vi "dataProcess_peaks_extended.vi"(0 "reference":refnum<class "OSA.lvclass">, 1 "X search full range":bool=TRUE, 7 "error in (no error)":errorcluster, 8 "X search min (/cm)":sgl format="%.2f", 9 "minPeakHeight (dB)":sgl format="%.2f", 12 "X search max (/cm)":sgl format="%.2f", 13 "thld (mW)":sgl format="%.2f", 15 "sorting (none)":enum16{"none", "position", "height", "width"}(ring)) -> (16 "peaks thld left":sgl[](array[numeric]), 17 "peakCenter centroid, (wavenr/cm)":sgl[](array[numeric]) format="%.2f", 18 "peaks thld right":sgl[](array[numeric]), 19 "peakHeight centroid, (mW power absolute)":sgl[](array[numeric]) format="%.2f", 20 "duplicate reference":refnum<class "OSA.lvclass">, 21 "nr peaksFound":i32, 23 "peak position, (wavenr/cm)":sgl[](array[numeric]) format="%.2f", 24 "peakWidth, (wavenr/cm)":sgl[](array[numeric]) format="%.2f", 25 "peakHeight, (mW power absolute)":sgl[](array[numeric]) format="%.2f", 27 "error out":errorcluster)   [LabVIEW 2010, in "OSA.lvclass"]
doc: "Make use of FTSLib FTS_FindPeaks_ext which enable a more detailed peaks characterisation, (centroid algorithm)."
uses:
  OSA.lvclass
  typeDef/spectrum_y_unit.ctl
  FTSLib.dll
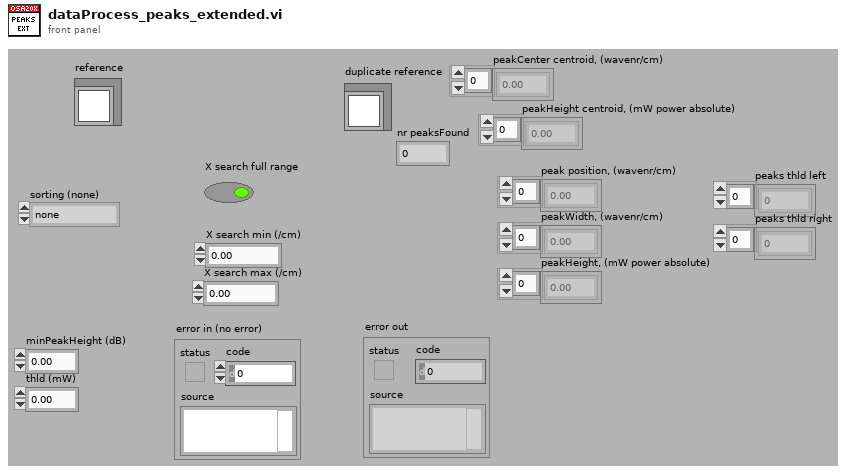
[diagram p1: front panel]
types:
  T1 = typedef "OSA.lvclass/spectrum_y_unit.ctl" = enum16{"dBm pwr absolute", "dBm pwr density", "mW pwr absolute", "mW pwr density"}
  T2 = enum16{"get", "init", "set interferogram", "set spectrum", "cleanUp"}
  T3 = typedef "OSA.lvclass/ObjectAttributes.ctl" = cluster{"Stop":bool, "dataType":T4, "spectrometerIdx":u16, "buffer size interferogram":i32, "interferogram":cluster{"new":bool, "plot_x_ min":sgl, "plot_x_max":sgl, "plot_y_min":sgl, "plot_y_max":sgl, "Graph Intrfrgrm":T5, "timeStamp":u32, "signal (%)":dbl, "traces":cluster{"idx":u32, "broadBand":bool, "monoChromatic":bool, "peakToPeakSignal":dbl, "peakToPeakPos":dbl}[], "traces idx last":i32}, "spectrum":cluster{"new":bool, "plot_x_min":sgl, "plot_x_max":sgl, "plot_unit_x":T6, "plot_unit_y":T7, "plot_y_min":sgl, "plot_y_max":sgl, "Graph Spectrum":T5, "timeStamp":u32, "X_VAL_OPTIONS":enum16{"MIN_MAX", "ARRAY"}, "traces":cluster{"idx":u32}[], "traces idx last":i32}, "Thorlabs_OSA_64.lvclass:queue_action.ctlqueue ref":refnum<queue>, "action":T8, "plot zoom step":dbl, "buffer semaphore":T9, "acq stopped":bool, "dataType active":T4, "temperature (degr C)":sgl, "pressure (hPa)":sgl, "rel humidity (%)":sgl, "settings":cluster{"resolution":T10, "sensitivity":T11, "Average":bool, "average nr":u32, "apodisation":T12, "acq delay (ms)":u32, "airMesure":T13, "wmtr on":bool, "intfgrm_smooth_width":u16, "intfgrm_smooth_nrOfPasses":u16, "intfgrm_smooth":T14, "phaseCorrection":T15, "zeroFill":u8, "spectr_smooth":T14, "spectr_smooth_width":u16, "spectr_smooth_nrOfPasses":u16, "resolution (/cm)":sgl, "REF wavelength, (nm)":dbl, "gain_idx":u16, "gainAuto":bool, "gain_relative":dbl, "PD sensitivity mode":T16, "PD senseMode implemented":bool, "SensorTemperature implemented":bool, "SensorPressure implemented":bool, "SensorHumidity implemented":bool}, "peaks position":sgl[], "peaks width":sgl[], "peaks height":sgl[], "peaks max nr":u32, "peaks latest nr":i32, "peaks new":bool, "power":dbl, "power new":bool, "path":string, "wavelength (WNr)":dbl, "wavelength new":bool, "buffer size spectrum":i32, "status":string, "VI reference":refnum<vi>, "funcPointer":u64, "libraryPointer":u64, "singleAcquisition":bool, "coherenceLength (cm)":dbl, "coherenceLength new":bool, "spectrometer model":string, "spectrometer serial nr":string, "peaks thld left":sgl[], "peaks thld right":sgl[], "coherenceLength error (cm)":dbl, "ADC bits":u16, "peaks position centroid":sgl[], "peaks height centroid":sgl[], "OSA series":T17, "channel index spectrum":u16, "spectrometer rangeLow, (/cm)":dbl, "spectrometer rangeHigh, (/cm)":dbl, "channel index interferogram":u16}
  T4 = typedef "OSA.lvclass/acq_dataType.ctl" = enum16{"none", "interferogram", "spectrum"}
  T5 = typedef "OSA.lvclass/graph_intensity.ctl" = refnum<vi>
  T6 = typedef "OSA.lvclass/spectrum_x_unit.ctl" = enum16{"wavenr/cm", "THz", "eV", "nm_air", "nm_vac"}
  T7 = typedef "OSA.lvclass/y_unit.ctl" = enum16{"ADC counts", "dBm pwr absolute", "dBm pwr density", "mW pwr absolute", "mW pwr density"}
  T8 = typedef "OSA.lvclass/queue_action.ctl" = enum16{"none", "stop", "GUI_plotInterferogram", "GUI_plotSpectrum", "GUI_plotInterferogramRescale", "GUI_plotSpectrumRescale", "GUI_plotInterferogramReset", "GUI_plotSpectrumReset", "GUI_plotInterferogramAutoScaleY", "GUI_plotSpectrumAutoScaleY", "GUI_plotInterferogramZoomOut", "GUI_plotSpectrumZoomOut", "GUI_plotInterferogramPane", "GUI_plotSpectrumPane", "GUI_plotInterferogramZoomMouse", "GUI_plotSpectrumZoomMouse", "ENVIRONMENT temperature", "ENVIRONMENT pressure", "MODE_resolution set", "MODE_resolution get", "MODE_sensitivity set", "MODE_sensitivity get", "MODE_PDTemperature set", "MODE_PDTemperature get", "REBOOT/RESET firmware", "ACQASYNC_acquireSingleSpectrum", "ACQASYNC_continuous start", "ACQASYNC_continuous stop\n", "ACQASYNC_get last interferogram", "ACQASYNC_get last spectrum", "ACQASYNC_get last waveNr", "ACQOPT_interferogram smoothing set", "ACQOPT_interferogram smoothing get", "ACQOPT_spectrum smoothing set", "ACQOPT_spectrum smoothing get", "ACQOPT_apodisation type set", "ACQOPT_apodisation type get", "ACQOPT_phase correction type set", "ACQOPT_phase correction type get", "ACQOPT_acqIntervall_set", "ACQOPT_acqIntervall_get", "ACQOPT_average spectrum set", "ACQOPT_average spectrum get", "ACQOPT_rolling average set", "ACQOPT_rolling average get", "ACQOPT_zero fill factor set", "ACQOPT_zero fill factor get", "ACQOPT_cycle counting set", "ACQOPT_cycle counting get", "ACQOPT_air measure option set", "ACQOPT_air measure option get", "ACQOPT_gainLevel auto get", "ACQOPT_gainLevel auto set", "ACQOPT_gainLevel get", "ACQOPT_gainLevel set", "ACQOPT_getAll", "INSTRUMENT_PROPERTY_range_WaveNr_min", "INSTRUMENT_PROPERTY_range_WaveNr_max", "INSTRUMENT_PROPERTY_reference_wavelength_cm^-1", "INSTRUMENT_PROPERTY_samplesPerRefPeriod", "INSTRUMENT_PROPERTY_resolution_waveNrPercm", "INSTRUMENT_PROPERTY_availableGainLevels", "INSTRUMENT_PROPERTY_status", "CONVERT", "ANALYSE_POWER", "ANALYSE_PEAKS", "ANALYSE_WAVELENGTH", "ANALYSE_SPECTRUM", "ANALYSE_INTERFEROGRAM", "ANALYSE_COHERENCE_LENGTH", "MATH", "MATH_power", "MATH_peaks", "FILE", "miscellaneous"}
  T9 = typedef "Semaphore RefNum" = refnum<k1>
  T10 = typedef "OSA.lvclass/resolution.ctl" = enum16{"low", "high"}
  T11 = typedef "OSA.lvclass/sensitivityMode.ctl" = enum16{"low", "low medium", "high medium", "high"}
  T12 = typedef "OSA.lvclass/apodisation.ctl" = enum16{"NONE", "NORTON_BEER_WEAK", "NORTON_BEER_MEDIUM", "NORTON_BEER_STRONG", "TRIANGULAR", "COSINE", "HANN", "HAMMING", "BLACKMANHARRIS3", "BLACKMANHARRIS4", "GAUSSIAN"}
  T13 = typedef "OSA.lvclass/airMeasure.ctl" = enum16{"TEMPERATURE", "PRESSURE"}
  T14 = typedef "OSA.lvclass/interferogram_smoothing.ctl" = enum16{"NONE", "BINOMIAL", "SAVITSKY_GOLAY", "FOURIER", "MOVING_AVERAGE", "GAUSSIAN"}
  T15 = typedef "OSA.lvclass/phaseCorrection.ctl" = enum16{"NONE", "MERTZ", "FORMAN", "MERTZ_FILE", "FORMAN_FILE", "FUTURE COMP."}
  T16 = typedef "OSA.lvclass/PDTemperatureMode.ctl" = enum16{"cool: better sensitivity/noise floor", "warm: extended wl range"}
  T17 = typedef "OSA.lvclass/OSA_series.ctl" = enum16{"OSA200", "OSA300", "UNKNOWN"}
  T18 = typedef "OSA20X.lvclass/xVal_option.ctl" = enum16{"MIN_MAX", "ARRAY"}
  T19 = cluster{"length":u32, "X min":sgl, "X max":sgl, "X_VAL_OPTIONS":T18}
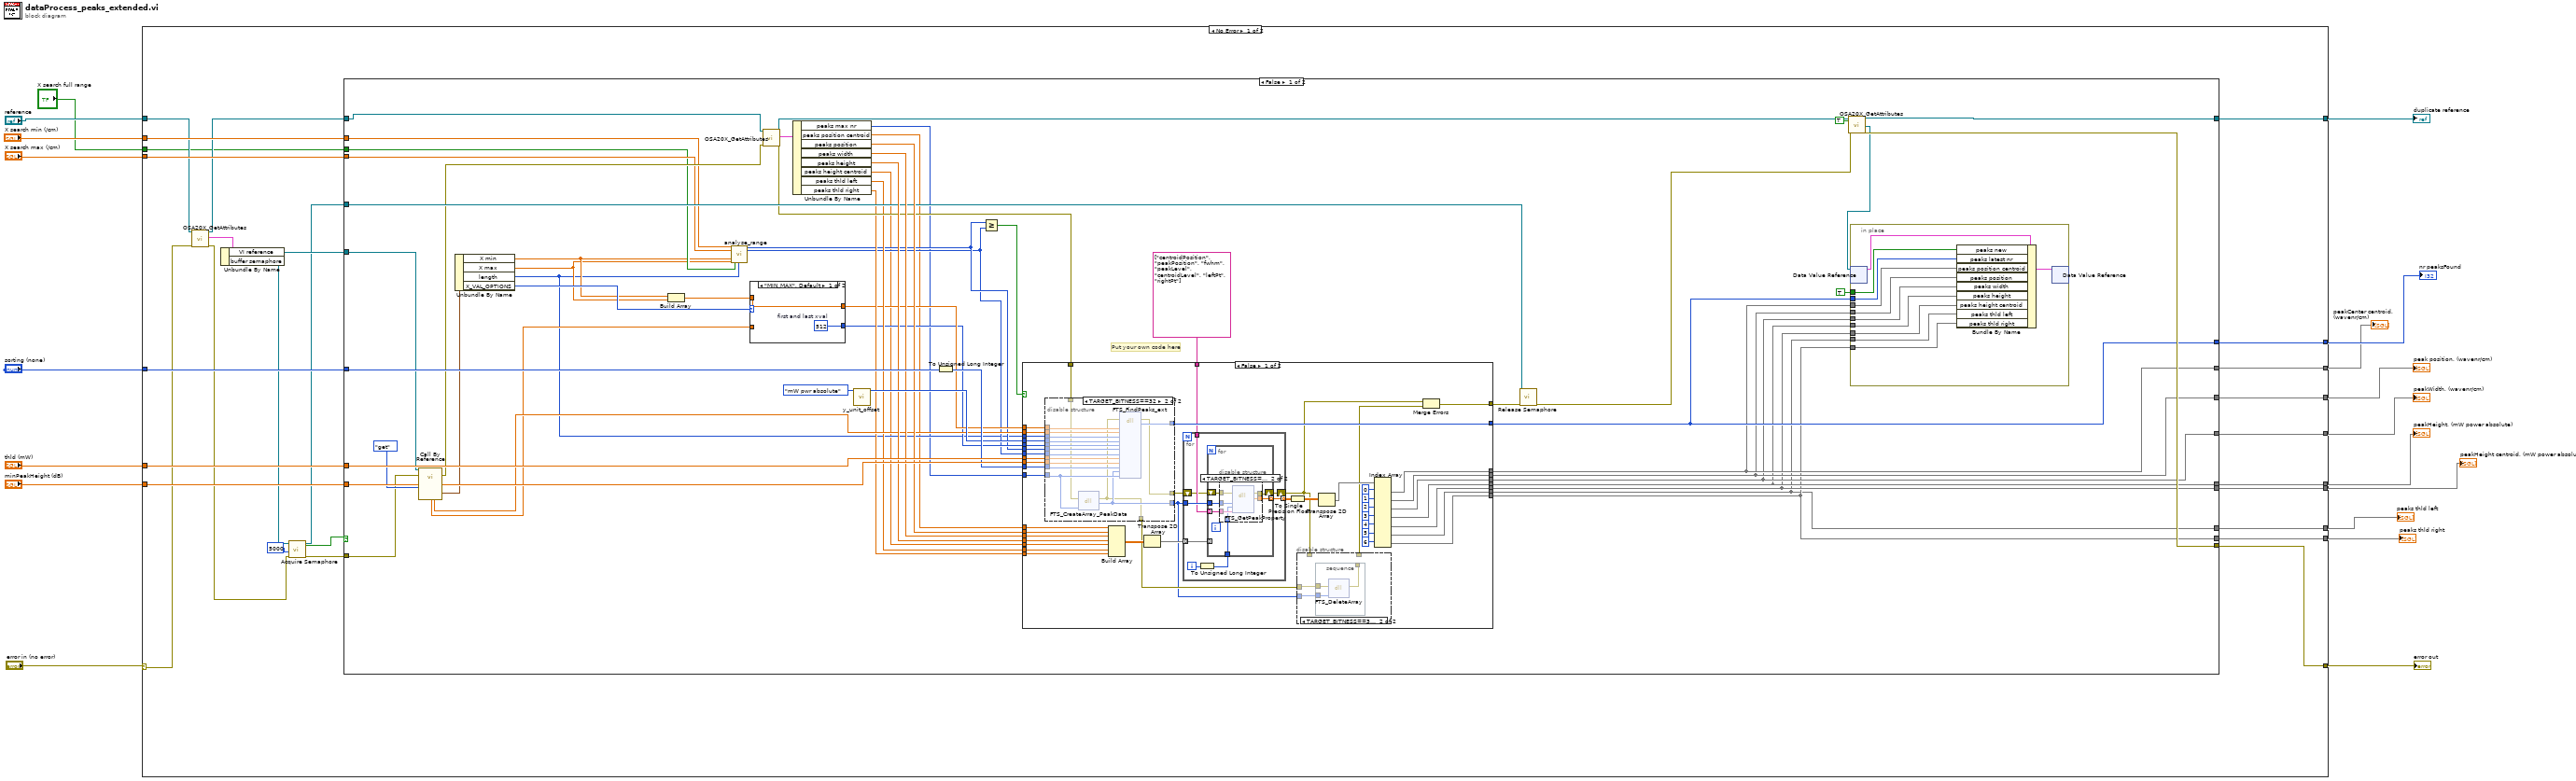
[diagram p0: block diagram]
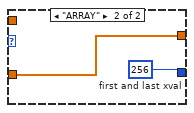
[diagram p2: hidden frame]
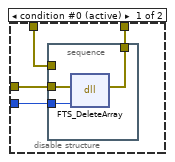
[diagram p3: hidden frame]
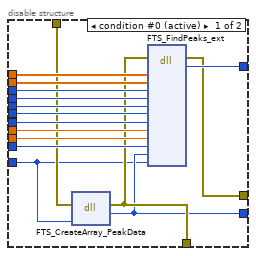
[diagram p4: hidden frame]
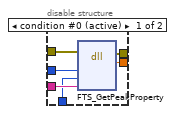
[diagram p5: hidden frame]
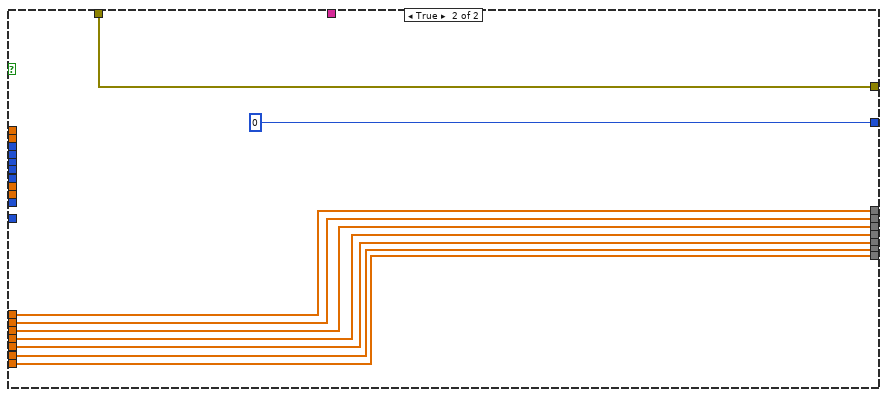
[diagram p6: hidden frame]
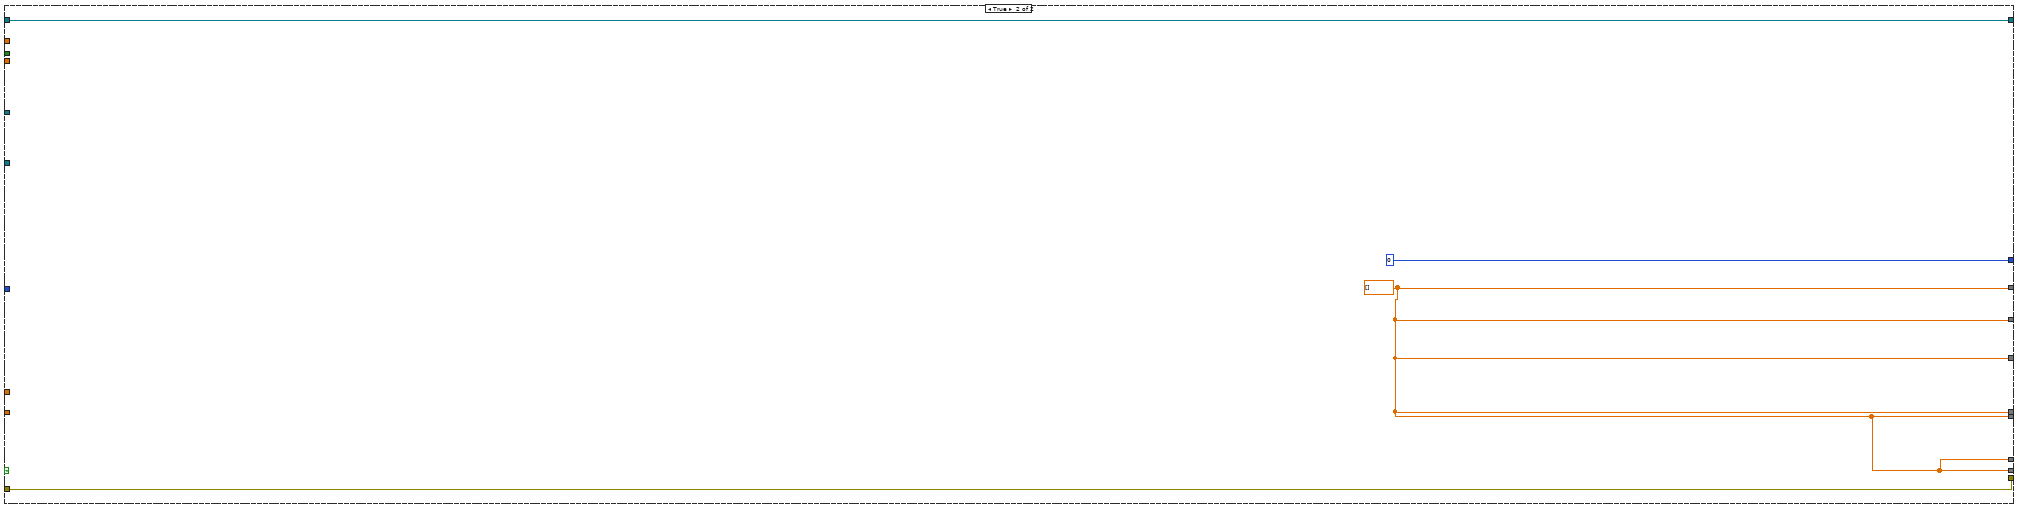
[diagram p7: hidden frame]
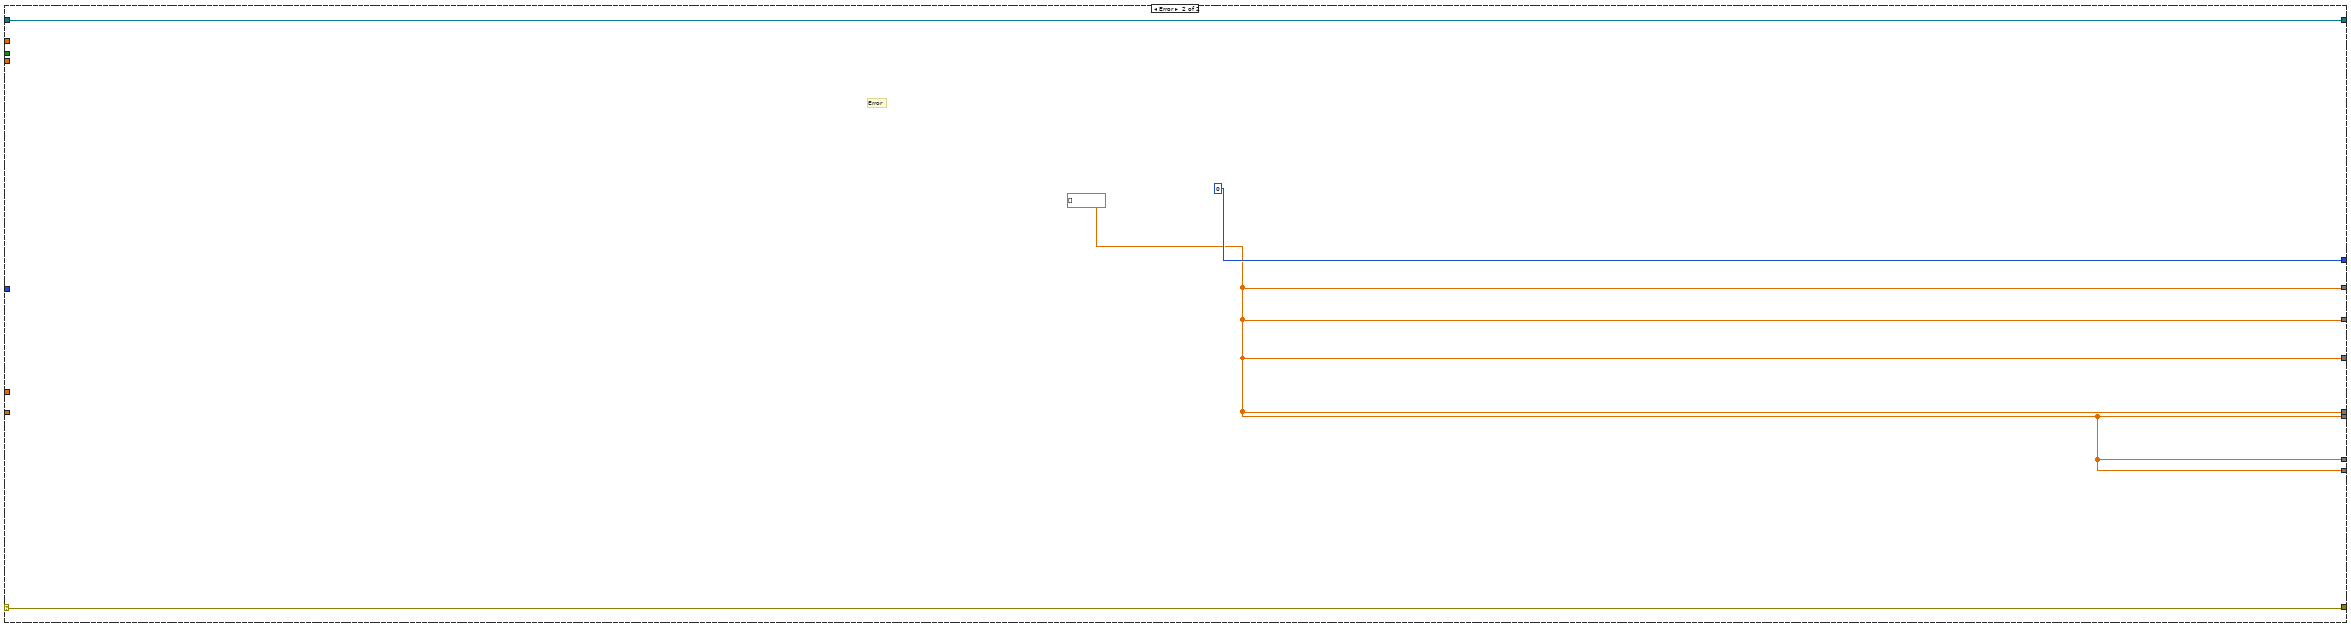
[diagram p8: hidden frame]
diagram:
  n1 = case shown="No Error" "error in (no error)" {
    selector: "error in (no error)" -> [w33 w247]
    tunnel: [w41 w247] -> w18
    tunnel: "reference" -> [w27 w248]
    tunnel: [w42 w248] -> w15
    tunnel: "minPeakHeight (dB)" -> [w45 _]
    tunnel: "thld (mW)" -> [w44 _]
    tunnel: "sorting (none)" -> [w43 _]
    tunnel: [w38 w245] -> w5
    tunnel: [w37 w245] -> w4
    tunnel: [w39 w245] -> w3
    tunnel: [w40 0] -> w11
    tunnel: "X search min (/cm)" -> [w36 _]
    tunnel: "X search max (/cm)" -> [w35 _]
    tunnel: [w23 w245] -> w2
    tunnel: [w22 w245] -> w1
    tunnel: "X search full range" -> [w21 _]
    tunnel: [w20 w245] -> w7
    tunnel: [w19 w245] -> w6
    frame No Error {
      n2 = call "OSA20X_GetAttributes.vi"("reference in"=w27, "error in (no error)"=w33) -> ("reference out"=w26:refnum<class "OSA.lvclass">, "Data"=w24:T3, "error out"=w32:errorcluster)  [unwired: 14 in, 1 out]
      n3 = Unbundle By Name(w24) -> ("VI reference"=w28:refnum<vi>, "buffer semaphore"=w30:T9)
      n4 = call <vilib>:"Acquire Semaphore.vi"("error in (no error)"=w32, "ms timeout (-1)"=5000, "semaphore"=w30) -> ("error out"=w31:errorcluster, "timed out"=w29:bool, "semaphore out"=w25:T9)  [unwired: 2 in]
      n5 = case shown="False" w29 {
        tunnel: w45 -> [w100 _]
        tunnel: w44 -> [w99 _]
        tunnel: w43 -> [w98 _]
        tunnel: w26 -> [w97 w243]
        tunnel: [w94 w243] -> w42
        tunnel: [w93 w242] -> w41
        tunnel: [w74 0 ("return type")] -> w40
        tunnel: [w71 w241] -> w39
        tunnel: [w73 w241] -> w38
        tunnel: [w72 w241] -> w37
        tunnel: w36 -> [w58 _]
        tunnel: w35 -> [w57 _]
        tunnel: w31 -> [w86 w242]
        tunnel: w28 -> [w85 _]
        tunnel: w25 -> [w80 _]
        tunnel: [w67 w241] -> w23
        tunnel: [w66 w241] -> w22
        tunnel: w21 -> [w56 _]
        tunnel: [w47 w241] -> w20
        tunnel: [w46 w241] -> w19
        frame False {
          # "Put your own code here"
          n6 = call-by-ref "?"(reference=w85, error in=w86, "action"=T2."get") -> (error out=w79:errorcluster, "spectrum X"=w64:sgl[], "spectrum Y"=w84:sgl[], "spectrum property"=w83:T19)  [unwired: 14 in, 3 out]
          n7 = Unbundle By Name(w83) -> ("X min"=w54:sgl, "X max"=w53:sgl, "length"=w52:u32, "X_VAL_OPTIONS"=w61:T18)
          n8 = Build Array(w54, w53) -> (w55:sgl[])
          n9 = call "analyse_range.vi"("X search min (/cm)"=w58, "X search max (/cm)"=w57, "X min"=w54, "X max"=w53, "full range"=w56, "length"=w52) -> ("index start"=w60:u32, "index stop"=w59:u32)  [unwired: 12 in]
          n10 = case shown="\"MIN_MAX\", Default" w61 {
            tunnel: w64 -> [_ w104]
            tunnel: [w102 w104] -> w63
            tunnel: w55 -> [w102 _]
            tunnel: [w101 w103] -> w62
            frame "MIN_MAX", Default {
              w101 = u32 512  # first and last xval
            }
            frame "ARRAY" {
              w103 = u32 256  # first and last xval
            }
          }
          n11 = call "OSA20X_GetAttributes.vi"("reference in"=w97, "error in (no error)"=w79) -> ("reference out"=w95:refnum<class "OSA.lvclass">, "Data"=w77:T3, "error out"=w70:errorcluster)  [unwired: 14 in, 1 out]
          n12 = Unbundle By Name(w77) -> ("peaks max nr"=w51:u32, "peaks position centroid"=w50:sgl[], "peaks position"=w90:sgl[], "peaks width"=w89:sgl[], "peaks height"=w88:sgl[], "peaks height centroid"=w49:sgl[], "peaks thld left"=w69:sgl[], "peaks thld right"=w68:sgl[])
          n13 = call "y_unit_offset.vi"("spectrum y unit (mW pwr absolute)"=spectrum_y_unit."mW pwr absolute") -> ("yUnit val"=w92:i32)  [unwired: 18 in]
          n14 = To Unsigned Long Integer(number=w98) -> (unsigned 32bit integer=w96:u32)
          n15 = Greater Or Equal?(x=w60, y=w59) -> (x >= y?=w91:bool)
          n16 = case shown="False" w91 {
            tunnel: w100 -> [w161 _]
            tunnel: w99 -> [w160 _]
            tunnel: w96 -> [w159 _]
            tunnel: w90 -> [w147 w237]
            tunnel: w89 -> [w146 w236]
            tunnel: w88 -> [w145 w235]
            tunnel: w51 -> [w116 _]
            tunnel: [w158 0] -> w74
            tunnel: w84 -> [w157 _]
            tunnel: [w135 w236] -> w71
            tunnel: [w137 w238] -> w73
            tunnel: [w136 w237] -> w72
            tunnel: w92 -> [w156 _]
            tunnel: w62 -> [w155 _]
            tunnel: w63 -> [w154 _]
            tunnel: w52 -> [w153 _]
            tunnel: w60 -> [w152 _]
            tunnel: w59 -> [w151 _]
            tunnel: [w119 w239] -> w82
            tunnel: w70 -> [w150 w239]
            tunnel: w69 -> [w143 w233]
            tunnel: w68 -> [w142 w232]
            tunnel: [w134 w235] -> w67
            tunnel: [w133 w234] -> w66
            tunnel: w50 -> [w148 w238]
            tunnel: w49 -> [w144 w234]
            tunnel: string[] ["centroidPosition", "peakPosition", "fwhm", "peakLevel", "centroidLevel", "leftPt", "rightPt"] -> [w149 _]
            tunnel: [w125 w233] -> w46
            tunnel: [w124 w232] -> w47
            frame False {
              n17 = disable-structure shown="TARGET_BITNESS==32" {
                disable-tunnel: w161 -> [w189 w197]
                disable-tunnel: w160 -> [w188 w198]
                disable-tunnel: w159 -> [w187 w196]
                disable-tunnel: [w186 w193] -> w158
                disable-tunnel: w157 -> [w185 w204]
                disable-tunnel: w156 -> [w184 w202]
                disable-tunnel: w155 -> [w183 w201]
                disable-tunnel: w154 -> [w182 w205]
                disable-tunnel: w153 -> [w181 w203]
                disable-tunnel: w152 -> [w180 w200]
                disable-tunnel: w151 -> [w179 w199]
                disable-tunnel: w150 -> [w178 w194]
                disable-tunnel: [w177 w192] -> w122
                disable-tunnel: [w176 w190] -> w121
                disable-tunnel: [w175 w191] -> w117
                disable-tunnel: w116 -> [w174 w195]
                frame condition #0 (active) {
                  n18 = dll-call lib="FTSLib.dll" fn="FTS_CreateArray_PeakData"(error in=w178, "number"=w174) -> (error out=w176:errorcluster, "return type"=w175:u64)  [unwired: 3 in, 1 out]
                  n19 = dll-call lib="FTSLib.dll" fn="FTS_FindPeaks_ext"(error in=w176, "xData"=w182, "yData"=w185, "length"=w181, "yAxisUnit"=w184, "xValueOption"=w183, "idxStart"=w180, "idxStop"=w179, "thld"=w188, "minPeakHeight_dB"=w189, "option"=w187, "peakArray"=w175, "maxPeaks"=w174) -> (error out=w177:errorcluster, "return type"=w186:i32)  [unwired: 14 in, 1 out]
                }
                frame condition #1 {
                  n20 = dll-call lib="FTSLib.dll" fn="FTS_CreateArray_PeakData"(error in=w194, "number"=w195) -> (error out=w190:errorcluster, "return type"=w191:u32)  [unwired: 3 in, 1 out]
                  n21 = dll-call lib="FTSLib.dll" fn="FTS_FindPeaks_ext"(error in=w190, "xData"=w205, "yData"=w204, "length"=w203, "yAxisUnit"=w202, "xValueOption"=w201, "idxStart"=w200, "idxStop"=w199, "thld"=w198, "minPeakHeight_dB"=w197, "option"=w196, "peakArray"=w191, "maxPeaks"=w195) -> (error out=w192:errorcluster, "return type"=w193:i32)  [unwired: 14 in, 1 out]
                }
              }
              n22 = Build Array(w148, w147, w146, w145, w144, w143, w142) -> (w141:sgl[][])
              n23 = Transpose 2D Array(2D array=w141) -> (transposed array=w140:sgl[][])
              n24 = for {
                tunnel: w117 -> [w213]
                tunnel: w149 -> [w212]
                tunnel: w140 -> [w211] mode=indexing
                tunnel: [w208] -> w139 mode=indexing
                shift-right: [w206] -> w118
                shift-left: w122 -> [w207]
                i -> [w210]
                n25 = To Unsigned Long Integer(number=w210) -> (unsigned 32bit integer=w209:u32)
                n26 = for {
                  tunnel: w213 -> [w219]
                  tunnel: w212 -> [w218] mode=indexing
                  tunnel: w211 -> [_] mode=indexing
                  tunnel: [w217] -> w208 mode=indexing
                  tunnel: w209 -> [w216]
                  shift-right: [w214] -> w206
                  shift-left: w207 -> [w215]
                  n27 = disable-structure shown="TARGET_BITNESS==32" {
                    disable-tunnel: w219 -> [w225 w231]
                    disable-tunnel: w218 -> [w224 w228]
                    disable-tunnel: [w223 w226] -> w217
                    disable-tunnel: w216 -> [w222 w227]
                    disable-tunnel: w215 -> [w221 w230]
                    disable-tunnel: [w220 w229] -> w214
                    frame condition #0 (active) {
                      n28 = dll-call lib="FTSLib.dll" fn="FTS_GetPeakProperty"(error in=w221, "peakArray"=w225, "indexOfPeak"=w222, "parameterName"=w224) -> (error out=w220:errorcluster, "return type"=w223:dbl)  [unwired: 5 in, 1 out]
                    }
                    frame condition #1 {
                      n29 = dll-call lib="FTSLib.dll" fn="FTS_GetPeakProperty"(error in=w230, "peakArray"=w231, "indexOfPeak"=w227, "parameterName"=w228) -> (error out=w229:errorcluster, "return type"=w226:dbl)  [unwired: 5 in, 1 out]
                    }
                  }
                }
              }
              n30 = To Single Precision Float(number=w139) -> (single precision float=w123:sgl[][])
              n31 = disable-structure shown="TARGET_BITNESS==32" {
                disable-tunnel: w121 -> [w165 w169]
                disable-tunnel: [w164 _] -> w120
                disable-tunnel: w118 -> [w163 _]
                disable-tunnel: w117 -> [w162 w170]
                frame condition #0 (active) {
                  n32 = stacked-sequence {
                    tunnel: w165 -> [w168]
                    tunnel: [w167] -> w164
                    tunnel: w163 -> [_]
                    tunnel: w162 -> [w166]
                    frame #0 {
                      n33 = dll-call lib="FTSLib.dll" fn="FTS_DeleteArray"(error in=w168, "number"=w166) -> (error out=w167:errorcluster)  [unwired: 4 in, 1 out]
                    }
                  }
                }
                frame condition #1 {
                  n34 = stacked-sequence {
                    tunnel: w169 -> [w173]
                    tunnel: [w172] -> _
                    tunnel: w170 -> [w171]
                    frame #0 {
                      n35 = dll-call lib="FTSLib.dll" fn="FTS_DeleteArray"(error in=w173, "number"=w171) -> (error out=w172:errorcluster)  [unwired: 4 in, 1 out]
                    }
                  }
                }
              }
              n36 = Transpose 2D Array(2D array=w123) -> (transposed array=w138:sgl[][])
              n37 = Index Array(array=w138, index (row) #1=0 ("index (row)"), index (row) #2=1 ("index (row)"), index (row) #3=2 ("index (row)"), index (row) #4=3 ("index (row)"), index (row) #5=4 ("index (row)"), index (row) #6=5 ("index (row)"), index (row) #7=6 ("index (row)")) -> (element #1=w137:sgl[], element #2=w136:sgl[], element #3=w135:sgl[], element #4=w134:sgl[], element #5=w133:sgl[], element #6=w125:sgl[], element #7=w124:sgl[])  [unwired: 7 in]
              n38 = Merge Errors(w118, w120) -> (w119:errorcluster)
            }
            frame True {
            }
          }
          n39 = call <vilib>:"Release Semaphore.vi"("error in (no error)"=w82, "semaphore"=w80) -> ("error out"=w81:errorcluster)  [unwired: 4 in, 1 out]
          n40 = call "OSA20X_GetAttributes.vi"("reference in"=w95, "OnlyGetDvrReference(False)"=TRUE, "error in (no error)"=w81) -> ("reference out"=w94:refnum<class "OSA.lvclass">, "DataRef"=w76:refnum<data-value>, "error out"=w93:errorcluster)  [unwired: 13 in, 1 out]
          n41 = in-place {
            in-place-border: TRUE ("peaks new") -> [w114]
            in-place-border: w74 -> [w113]
            in-place-border: w73 -> [w112]
            in-place-border: w72 -> [w110]
            in-place-border: w71 -> [w109]
            in-place-border: w67 -> [w108]
            in-place-border: w66 -> [w107]
            in-place-border: w46 -> [w106]
            in-place-border: w47 -> [w105]
            n42 = in-place-dvr #1(w76) -> (w115:T3)  [unwired: 1 out]
            n43 = Bundle By Name(cluster=w115, "peaks new"=w114, "peaks latest nr"=w113, "peaks position centroid"=w112, "peaks position"=w110, "peaks width"=w109, "peaks height"=w108, "peaks height centroid"=w107, "peaks thld left"=w106, "peaks thld right"=w105) -> (w111:T3)
            n44 = in-place-dvr #1(w111) -> ()  [unwired: 2 out]
          }
        }
        frame True {
          w241 = sgl[] [] ("peaks position")
        }
      }
    }
    frame Error {
      w245 = sgl[] [] ("peakCenter")
      # "Error"
    }
  }
  "error out" <- w18
  "duplicate reference" <- w15
  "peak position, (wavenr/cm)" <- w4
  "peakWidth, (wavenr/cm)" <- w3
  "peakHeight, (mW power absolute)" <- w2
  "nr peaksFound" <- w11
  "peaks thld left" <- w6
  "peaks thld right" <- w7
  "peakCenter centroid, (wavenr/cm)" <- w5
  "peakHeight centroid, (mW power absolute)" <- w1
